vi "SetBackground.vi"(8 "error in (no error)":errorcluster, 11 "Bouncer in":refnum<class "Bouncer.lvclass">) -> (0 "error out":errorcluster, 3 "Bouncer out":refnum<class "Bouncer.lvclass">)   [LabVIEW 2019, in "RT_Game.lvlib" / "Bouncer.lvclass"]
uses:
  Bouncer.lvclass
  C:/Users/FreshBob/Dropbox/VIs/myRIO_GameConsole/RT/RT_Game/Game/Game.lvclass
  Game/Coordinate.ctl
  Game/Game.lvclass
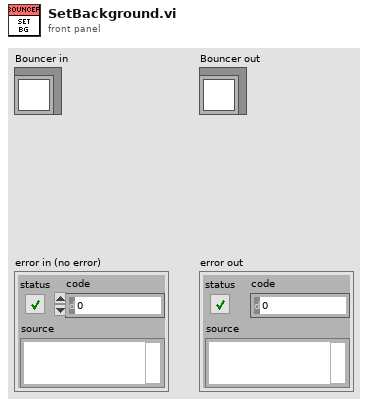
[diagram p1: front panel]
types:
  T1 = typedef "RT_Game.lvlib/Game.lvclass/Coordinate.ctl" = cluster{"x":dbl, "y":dbl}
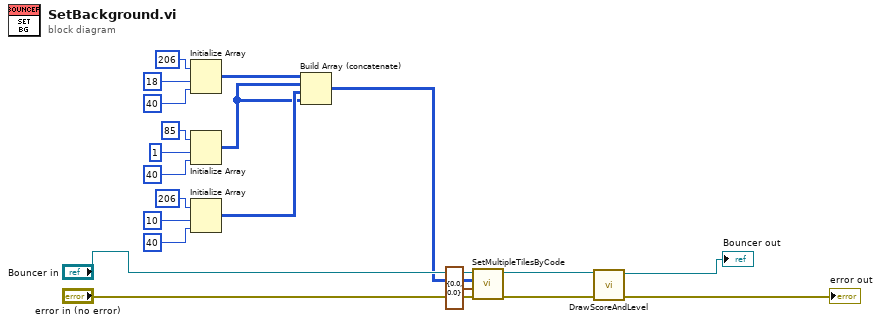
[diagram p0: block diagram]
diagram:
  n1 = Initialize Array(u16 206 ("dimension size"), 18 ("dimension size"), 40 ("dimension size")) -> (w20:u16[][])
  n2 = Initialize Array(u16 85 ("dimension size"), 1 ("dimension size"), 40 ("dimension size")) -> (w5:u16[][])
  n3 = Initialize Array(u16 206 ("dimension size"), 10 ("dimension size"), 40 ("dimension size")) -> (w6:u16[][])
  n4 = Build Array (concatenate)(w20, w5, w6, w5) -> (w10:u16[][])
  n5 = call "SetMultipleTilesByCode.vi"("error in (no error)"="error in (no error)", "Position"=T1 {"x"=0.0, "y"=0.0}, "TileCodes"=w10, "Game in"="Bouncer in") -> ("error out"=w15:errorcluster, "Game out"=w1:refnum<class "Bouncer.lvclass">)  [unwired: 6 in]
  n6 = call "DrawScoreAndLevel.vi"("error in (no error)"=w15, "Bouncer in"=w1) -> ("error out"=→"error out":errorcluster, "Bouncer out"=→"Bouncer out":refnum<class "Bouncer.lvclass">)  [unwired: 8 in]
